vi "fetchData.vi"   [LabVIEW 2017]
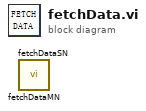
[diagram p0: block diagram]
diagram:
  n1 = call "fetchDataMN.vi"() -> ()  [unwired: 10 in, 2 out]
  n2 = call "fetchDataSN.vi"() -> ()  [unwired: 12 in]
